vi "Configure Measurement.vi"(0 "Supply Handle in":refnum<k15>, 1 "Channel Name(s)":string, 5 "Measurement Configuration":T1={"Measure When Mode"=1027, "Sense Mode"=1008, "Measurement Trigger Terminal"="PXI_Trig0", "Measurement Mode"=enum."Single Point", "Measurement Time (s)"=0.001} {"Measure When Mode" items=["Automatically after Source Complete"=1025, "On Demand"=1026, "On Measure Trigger"=1027]; "Sense Mode" items=["Local"=1008, "Remote"=1009]; "Measurement Time (s)" format="%#_13p"}, 11 "error in (no error)":errorcluster) -> (4 "Supply Handle out":refnum<k15>, 15 "error out":errorcluster)   [LabVIEW 2019, in "Supply.lvlib"]
uses:
  Supply.lvlib
  Typedefs/Measurement Configuration.ctl
  <instrlib>/niDCPower/nidcpower.llb/niDCPower Sense.ctl
  <instrlib>/niDCPower/nidcpower.llb/niDCPower Configure Digital Edge Measure Trigger.vi
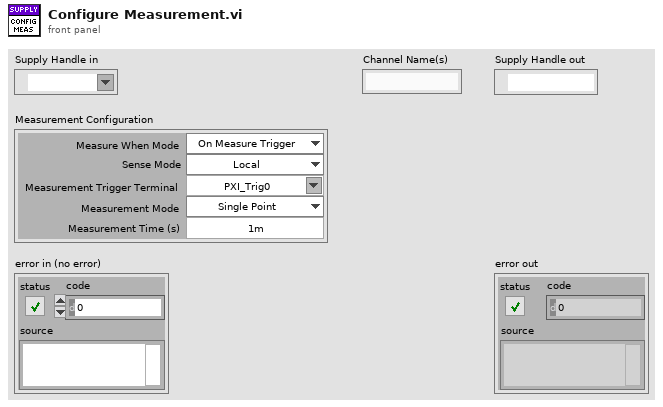
[diagram p1: front panel]
types:
  T1 = typedef "Supply.lvlib/Measurement Configuration.ctl" = cluster{"Measure When Mode":i32, "Sense Mode":T2, "Measurement Trigger Terminal":string, "Measurement Mode":enum16{"Single Point", "Record"}, "Measurement Time (s)":dbl}
  T2 = typedef "niDCPower Sense.ctl" = i32
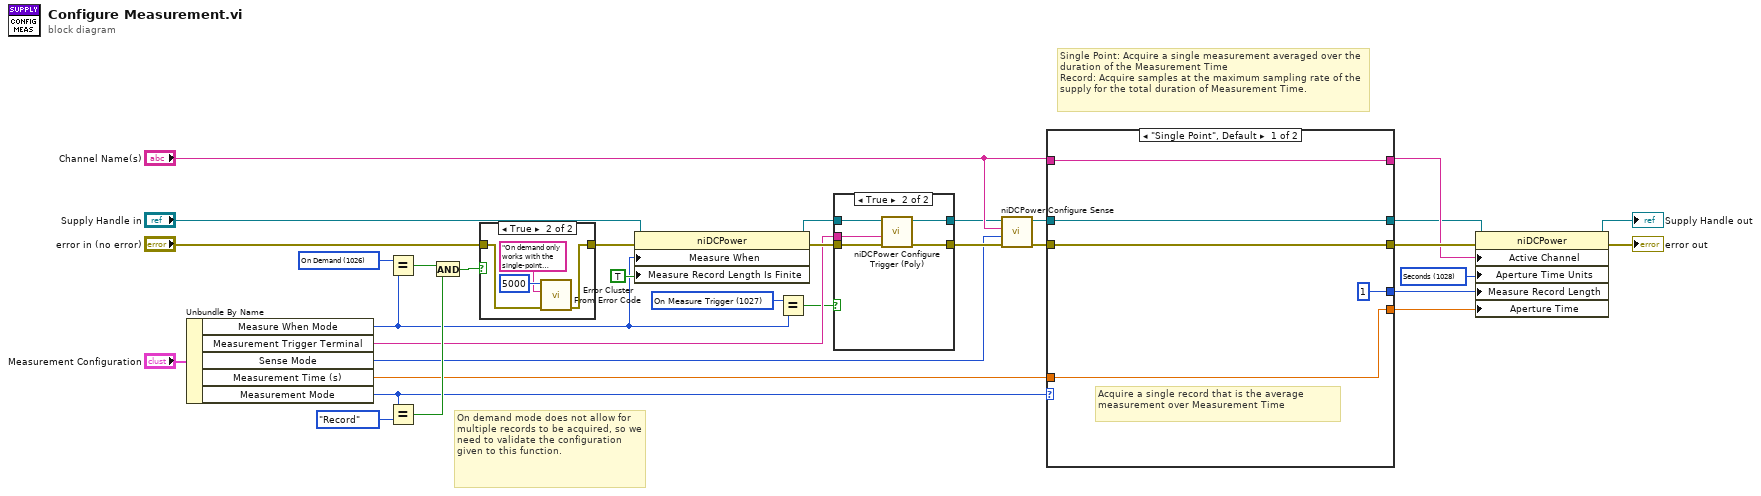
[diagram p0: block diagram]
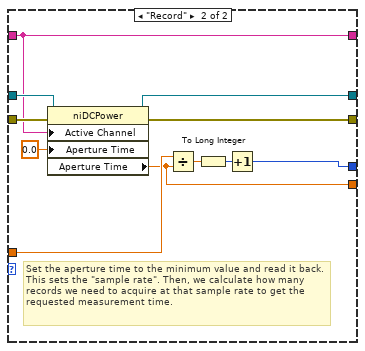
[diagram p4: hidden frame]
diagram:
  w3 = 1027 items=["Automatically after Source Complete"=1025, "On Demand"=1026, "On Measure Trigger"=1027] ("Measurement:Advanced:Measure When")
  w4 = 1026 items=["Automatically after Source Complete"=1025, "On Demand"=1026, "On Measure Trigger"=1027] ("Measurement:Advanced:Measure When")
  w26 = 1028 items=["Seconds"=1028, "Power Line Cycles"=1029] ("Measurement:Aperture Time Units")
  # "Single Point: Acquire a single measurement averaged over the duration of the Measurement Time\nRecord: Acquire samples at the maximum sampling rate of the supply for the total duration of Measurement Time."
  # "On demand mode does not allow for multiple records to be acquired, so we need to validate the configuration given to this function."
  n1 = Unbundle By Name("Measurement Configuration") -> ("Measure When Mode"=w2:i32, "Measurement Trigger Terminal"=w6:string, "Sense Mode"=w5:T2, "Measurement Time (s)"=w28:dbl, "Measurement Mode"=w18:enum16{"Single Point", "Record"})
  n2 = Equal?(x=w4, y=w2) -> (x = y?=w16:bool)
  n3 = Equal?(x=w18, y=enum16{"Single Point", "Record"}."Record" ("Measurement Mode")) -> (x = y?=w32:bool)
  n4 = And(x=w16, y=w32) -> (x .and. y?=w15:bool)
  n5 = case shown="True" w15 {
    tunnel: "error in (no error)" -> [w33 w35]
    tunnel: [w33 w34] -> w11
    frame False {
    }
    frame True {
      n6 = call <vilib>:"Error Cluster From Error Code.vi"("error in (no error)"=w35, "error message (\"\")"="On demand only works with the single-point measurement mode.", "error code (0)"=5000) -> ("error out"=w34:errorcluster)  [unwired: 6 in]
    }
  }
  n7 = property class="niDCPower"(reference="Supply Handle in", error in=w11, "Measure When"=w2, "Measure Record Length Is Finite"=TRUE ("Measurement:Measure Record Length Is Finite")) -> (reference out=w12:refnum<k15>, error out=w9:errorcluster)
  n8 = Equal?(x=w3, y=w2) -> (x = y?=w1:bool)
  n9 = case shown="True" w1 {
    tunnel: [w39 w44] -> w7
    tunnel: w12 -> [w39 w43]
    tunnel: w9 -> [w38 w42]
    tunnel: [w38 w41] -> w8
    tunnel: w6 -> [_ w40]
    frame False {
    }
    frame True {
      n10 = call-poly <instrlib>:"niDCPower Configure Trigger (Poly).vi"("error in (no error)"=w42, "input terminal"=w40, "instrument handle"=w43) -> ("error out"=w41:errorcluster, "instrument handle out"=w44:refnum<k15>)  [unwired: 7 in]
    }
  }
  n11 = call <instrlib>:"niDCPower Configure Sense.vi"("error in (no error)"=w8, "sense"=w5, "channel name"="Channel Name(s)", "instrument handle"=w7) -> ("error out"=w27:errorcluster, "instrument handle out"=w30:refnum<k15>)  [unwired: 6 in]
  n12 = case shown="\"Single Point\", Default" w18 {
    tunnel: w30 -> [w46 w55]
    tunnel: "Channel Name(s)" -> [w45 w51]
    tunnel: w28 -> [w49 w57]
    tunnel: w27 -> [w47 w56]
    tunnel: [w49 w50] -> w25
    tunnel: [1 ("Measurement:Measure Record Length") w54] -> w24
    tunnel: [w47 w53] -> w23
    tunnel: [w46 w52] -> w19
    tunnel: [w45 w51] -> w20
    frame "Single Point", Default {
      # "Acquire a single record that is the average measurement over Measurement Time"
    }
    frame "Record" {
      # "Set the aperture time to the minimum value and read it back. This sets the \"sample rate\". Then, we calculate how many records we need to acquire at that sample rate to get the requested measurement time."
      n13 = property class="niDCPower"(reference=w55, error in=w56, "Active Channel"=w51, "Aperture Time"=0.0 ("Measurement:Aperture Time")) -> (reference out=w52:refnum<k15>, error out=w53:errorcluster, "Aperture Time"=w50:dbl)
      n14 = Divide(x=w57, y=w50) -> (x/y=w60:dbl)
      n15 = To Long Integer(number=w60) -> (32bit integer=w59:i32)
      n16 = Increment(x=w59) -> (x+1=w54:i32)
    }
  }
  n17 = property class="niDCPower"(reference=w19, error in=w23, "Active Channel"=w20, "Aperture Time Units"=w26, "Measure Record Length"=w24, "Aperture Time"=w25) -> (reference out=→"Supply Handle out":refnum<k15>, error out=→"error out":errorcluster)
